vi "18.Evd.6_Ask.4.vi"() -> ()   [LabVIEW 2025]
panel:
  out "Average Temperature":dbl
  in  "Slide":dbl(slide) scale=0.0..10.0
  out "Number of Table Elements":dbl
  out "Repetition value per 1 sec":dbl[](array[numeric])
  in  "stop 2":bool
  in  "stop":bool
  out "Thermometer":dbl(slide) scale=0.0..100.0
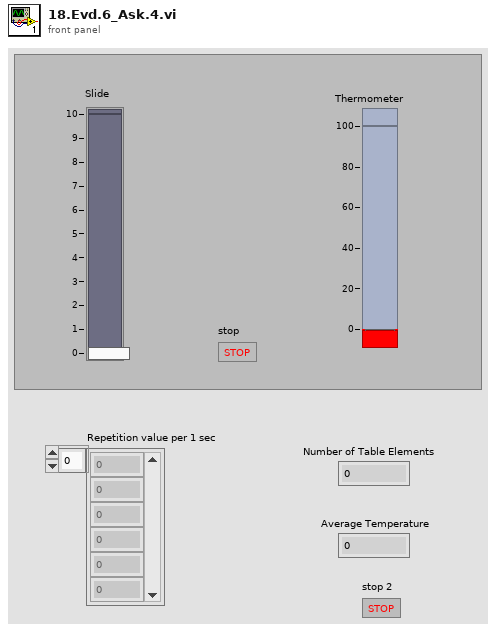
[diagram p1: front panel]
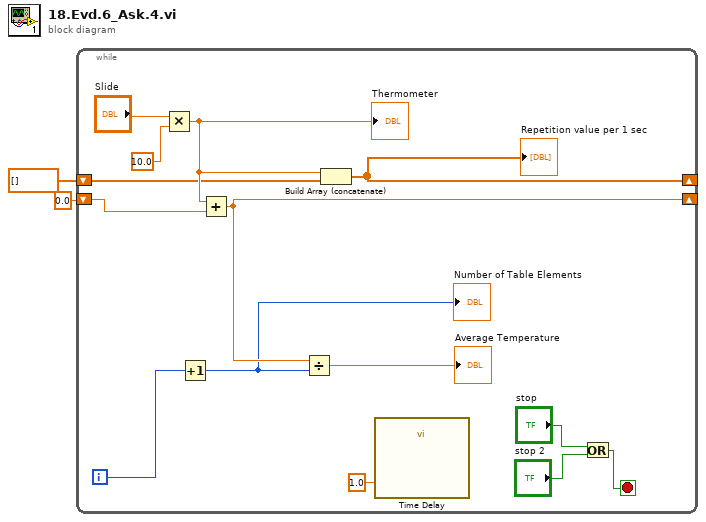
[diagram p0: block diagram]
diagram:
  n1 = while {
    shift-right: [w10] -> _
    shift-left: 0.0 -> [w11]
    shift-right: [w5] -> _
    shift-left: dbl[] [] -> [w8]
    i -> [w7]
    stop <- w14 stop-if-true
    n2 = Multiply(x="Slide", y=10.0) -> (x*y=w9:dbl)
    "Thermometer" <- w9
    n3 = Increment(x=w7) -> (x+1=w6:i32)
    "Number of Table Elements" <- w6
    n4 = Add(x=w9, y=w11) -> (x+y=w10:dbl)
    n5 = Divide(x=w10, y=w6) -> (x/y=→"Average Temperature":dbl)
    n6 = Build Array (concatenate)(w9, w8) -> (w5:dbl[])
    "Repetition value per 1 sec" <- w5
    n7 = call "Time Delay"("Delay Time (s)"=1.0) -> ()  [unwired: 10 in, 1 out]
    n8 = Or(x="stop", y="stop 2") -> (x .or. y?=w14:bool)
  }
